vi "get pid settings.vi"(8 "error in (no error)":errorcluster, 10 "pid_settings":T1, 11 "id":i32) -> (0 "error out":errorcluster, 2 "pid_settings out":T1, 3 "function return":i32)   [LabVIEW 2012, in "libximc.lvlib"]
doc: "result_t XIMC_API get_pid_settings (device_t id, pid_settings_t* pid_settings);"
uses:
  libximc.lvlib
  libximc.dll
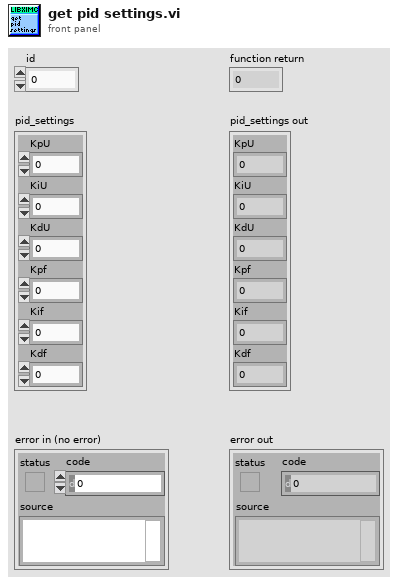
[diagram p1: front panel]
types:
  T1 = cluster{"KpU":u32, "KiU":u32, "KdU":u32, "Kpf":sgl, "Kif":sgl, "Kdf":sgl}
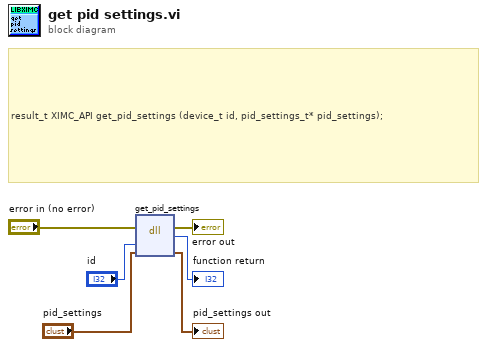
[diagram p0: block diagram]
diagram:
  # "result_t XIMC_API get_pid_settings (device_t id, pid_settings_t* pid_settings);"
  n1 = dll-call lib="C:/Users/Vasily/Att_examples/LabVIEW_example/libximc.*" fn="get_pid_settings"(error in="error in (no error)", "id"="id", "pid_settings"="pid_settings") -> (error out=→"error out":errorcluster, →"function return":i32, "pid_settings"=→"pid_settings out":T1)  [unwired: 3 in, 1 out]
